vi "ErrorHandler.vi"(8 "error in (no error)":errorcluster, 10 "Message (Error)":string="Error", 11 "ModuleAdmin In":refnum<class "ModuleAdmin.lvclass">) -> (0 "error out":errorcluster, 3 "ModuleAdmin Out":refnum<class "ModuleAdmin.lvclass">)   [LabVIEW 2018, in "AnalysisModule.lvlib"]
uses:
  AnalysisModule.lvlib
  <userlib>/NIST/ModuleAdminLib/ModuleAdmin/ModuleAdmin.lvclass
  <userlib>/NIST/ModuleAdminLib/ModuleAdmin/TypeDefinitions/QueueEntry.ctl
  <userlib>/NIST/ModuleAdminLib/ModuleAdmin/TypeDefinitions/QueueType.ctl
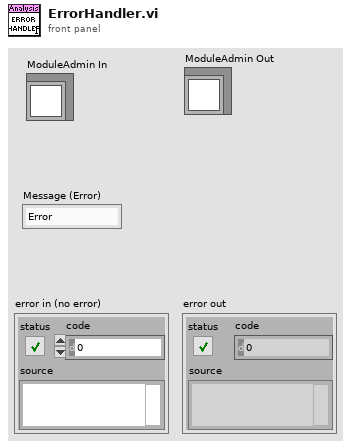
[diagram p1: front panel]
types:
  T1 = typedef "ModuleAdmin.lvlib/ModuleAdmin.lvclass/QueueType.ctl" = enum16{"EnqueueAtFront", "Enqueue", "Lossy Enqueue"}
  T2 = typedef "ModuleAdmin.lvlib/ModuleAdmin.lvclass/QueueEntry.ctl" = enum16{"QMH", "Class Data", "Data Loop", "Queue 4", "Queue 5", "Queue 6", "Queue 7", "Queue 8", "Queue 9", "Queue 10"}
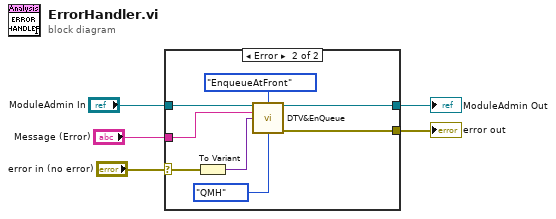
[diagram p0: block diagram]
diagram:
  n1 = case shown="Error" "error in (no error)" {
    selector: "error in (no error)" -> [w6 w15]
    tunnel: "Message (Error)" -> [_ w12]
    tunnel: [w7 w14] -> w3
    tunnel: "ModuleAdmin In" -> [w7 w13]
    tunnel: [w6 w9] -> w1
    frame No Error {
    }
    frame Error {
      n2 = To Variant(anything=w15) -> (Variant=w11:variant)
      n3 = call "DTV&EnQueue.vi"("ModuleAdmin In"=w13, "Enqueue Type (Enqueue)"=QueueType."EnqueueAtFront", "Message"=w12, "Message Data"=w11, "QueueArrayEntry(QMH)"=QueueEntry."QMH") -> ("ModuleAdmin Out"=w14:refnum<class "ModuleAdmin.lvclass">, "Error Out"=w9:errorcluster)  [unwired: 7 in, 2 out]
    }
  }
  "error out" <- w1
  "ModuleAdmin Out" <- w3
